vi "Get SLSC Modules.vi"(8 "error in (no error)":errorcluster, 11 "SLSC Chassis":refnum<k24>) -> (0 "error out":errorcluster, 2 "SLSC Modules":refnum<k24>[](array[refnum]), 3 "SLSC Chassis out":refnum<k24>)   [LabVIEW 2019, in "VeriStand SLSC Scripting.lvlib"]
uses:
  VeriStand SLSC Scripting.lvlib
  NationalInstruments.VeriStand.SystemDefinitionAPI
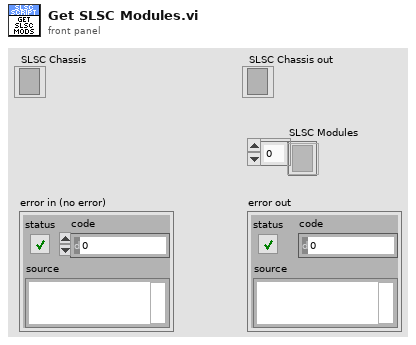
[diagram p1: front panel]
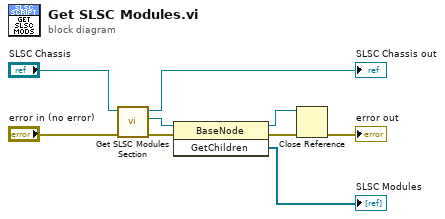
[diagram p0: block diagram]
diagram:
  n1 = call "Get SLSC Modules Section.vi"("error in (no error)"="error in (no error)", "SLSC Chassis"="SLSC Chassis") -> ("error out"=w2:errorcluster, "Modules Section"=w4:refnum<k24>, "SLSC Chassis out"=→"SLSC Chassis out":refnum<k24>)  [unwired: 7 in]
  n2 = invoke class="BaseNode" method="GetChildren"(reference=w4, error in=w2) -> (reference out=w1:refnum<k24>, error out=w9:errorcluster, "GetChildren"=→"SLSC Modules":refnum<k24>[])  [unwired: 1 in]
  n3 = Close Reference(reference=w1, error in (no error)=w9) -> (error out=→"error out":errorcluster)
